vi "FindTopAndBottomEdges (SubVI).vi"(0 "Calibrated Image Array":T3[](array[typedef]), 1 "Fit Options":T7={"Number of Lines"=1, "Type"=enum."First Edge Rake", "Min. Score"=10.0, "Max. Score"=1000.0, "Orientation"=0.0, "Angle Range"=45.0, "Angle Tolerance"=1.0, "Step Size"=196, "Min. SNR (db)"=0.0, "Min. Points (%)"=25.0, "Hough Iterations"=5} {"Min. Points (%)" min=0.0 max=100.0; "Min. SNR (db)" min=0.0; "Max. Score" min=0.0 max=1024.0; "Min. Score" min=0.0 max=1024.0 step=1.0}, 5 "Options: Top Edge Search":T6={"Search Direction"=2, "Edge Options"={"Edge Polarity"=0, "Kernel Size"=5, "Width"=3, "Minimum Edge Strength"=16.0, "Interpolation Type"=enum."Bilinear Fixed", "Data Processing Method"=enum."Average"}, "Show Search Area"=TRUE, "Show Search Lines"=TRUE, "Show Edges Found"=TRUE, "Show Result"=TRUE, "Search Area Color"=65280, "Search Lines Color"=255, "Edge Locations Color"=16776960, "Result Color"=16711680, "Overlay Group Name"=""} {"Search Direction" items=["Left to Right", "Right to Left", "Top to Bottom", "Bottom to Top"]; "Edge Options"."Edge Polarity" items=["All Edges", "Rising Edges", "Falling Edges"]; "Edge Options"."Minimum Edge Strength" format="%.2f"; "Edge Options"."Width" step=2; "Edge Options"."Kernel Size" step=2}, 9 "Options: Bottom Edge Search":T6={"Search Direction"=3, "Edge Options"={"Edge Polarity"=2, "Kernel Size"=9, "Width"=3, "Minimum Edge Strength"=17.0, "Interpolation Type"=enum."Bilinear Fixed", "Data Processing Method"=enum."Average"}, "Show Search Area"=TRUE, "Show Search Lines"=TRUE, "Show Edges Found"=TRUE, "Show Result"=TRUE, "Search Area Color"=65280, "Search Lines Color"=255, "Edge Locations Color"=16776960, "Result Color"=16711680, "Overlay Group Name"=""} {"Search Direction" items=["Left to Right", "Right to Left", "Top to Bottom", "Bottom to Top"]; "Edge Options"."Edge Polarity" items=["All Edges", "Rising Edges", "Falling Edges"]; "Edge Options"."Minimum Edge Strength" format="%.2f"; "Edge Options"."Width" step=2; "Edge Options"."Kernel Size" step=2}, 11 "error in (no error)":errorcluster) -> (4 "Analyzed Image Array":T3[](array[typedef]), 6 "Top Edges":T1(array[cluster]), 8 "Bottom Edges":T1(array[cluster]), 10 "Array of Edge Endpoint Arrays":sgl[][][](array[numeric]), 15 "error out":errorcluster)   [LabVIEW 2016]
uses:
  <vilib>/vision/Measure.llb/Straight Edge Options.ctl
  <vilib>/vision/Measure.llb/Straight Edge Process.ctl
  <vilib>/vision/Measure.llb/Edge Options.ctl
  <vilib>/vision/Measure.llb/Edge Polarity.ctl
  <vilib>/vision/Image Controls.llb/IMAQ Image.ctl
  <vilib>/vision/NI_Vision_Development_Module.lvlib
panel:
  in  "ROI Descriptor - BOTTOM":T2={"Global Rectangle"=[0, 898, 2592, 1846], "Contours"=[{"ID"=enum."External", "Type"=12, "Coordinates"=[2, 898, 2591, 1846, 0]}]} {"Contours"."Type" items=["No Selection", "Point", "Line", "Rectangle", "Oval", "Polygon", "Freehand Region", "Annulus", "Unused2", "Unused3", "Broken Line", "Freehand Line", "Rotated Rectangle"]}
  in  "ROI Descriptor - TOP":T2={"Global Rectangle"=[0, 132, 2592, 1180], "Contours"=[{"ID"=enum."External", "Type"=12, "Coordinates"=[5, 132, 2612, 1180, 0]}]} {"Contours"."Type" items=["No Selection", "Point", "Line", "Rectangle", "Oval", "Polygon", "Freehand Region", "Annulus", "Unused2", "Unused3", "Broken Line", "Freehand Line", "Rotated Rectangle"]}
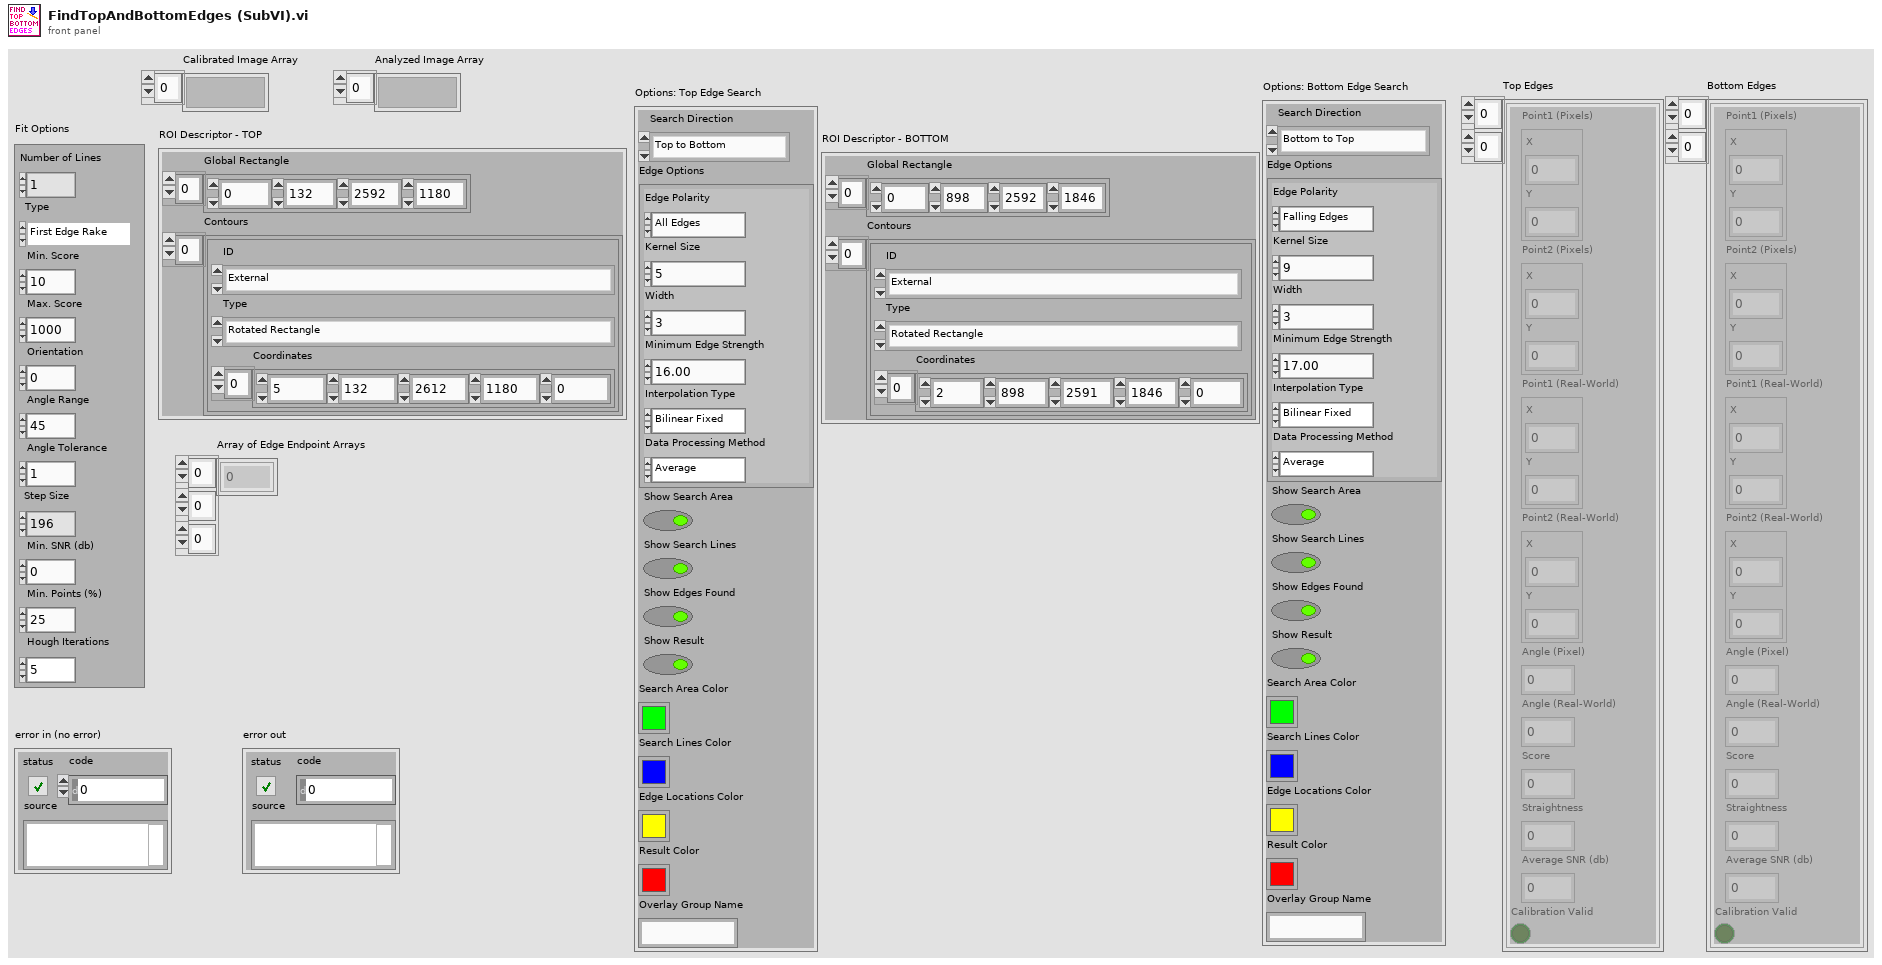
[diagram p1: front panel]
types:
  T1 = cluster{"Point1 (Pixels)":cluster{"X":sgl, "Y":sgl}, "Point2 (Pixels)":cluster{"X":sgl, "Y":sgl}, "Point1 (Real-World)":cluster{"X":sgl, "Y":sgl}, "Point2 (Real-World)":cluster{"X":sgl, "Y":sgl}, "Angle (Pixel)":dbl, "Angle (Real-World)":dbl, "Score":dbl, "Straightness":dbl, "Average SNR (db)":dbl, "Calibration Valid":bool}[][]
  T2 = cluster{"Global Rectangle":i32[], "Contours":cluster{"ID":enum32{"External", "Internal"}, "Type":u32, "Coordinates":i32[]}[]}
  T3 = typedef "IMAQ Image.ctl" = refnum<image>
  T4 = typedef "Edge Options.ctl" = cluster{"Edge Polarity":T5, "Kernel Size":u32, "Width":u32, "Minimum Edge Strength":sgl, "Interpolation Type":enum32{"Zero Order", "Bilinear", "Quadratic", "Cubic", "Bilinear Fixed"}, "Data Processing Method":enum32{"Average", "Median"}}
  T5 = typedef "Edge Polarity.ctl" = u32
  T6 = cluster{"Search Direction":u32, "Edge Options":T4, "Show Search Area":bool, "Show Search Lines":bool, "Show Edges Found":bool, "Show Result":bool, "Search Area Color":u32, "Search Lines Color":u32, "Edge Locations Color":u32, "Result Color":u32, "Overlay Group Name":string}
  T7 = typedef "Straight Edge Options.ctl" = cluster{"Number of Lines":i32, "Type":T8, "Min. Score":dbl, "Max. Score":dbl, "Orientation":dbl, "Angle Range":dbl, "Angle Tolerance":dbl, "Step Size":u32, "Min. SNR (db)":dbl, "Min. Points (%)":dbl, "Hough Iterations":i32}
  T8 = typedef "Straight Edge Process.ctl" = enum32{"First Edge Rake", "Best Edge Rake", "Hough Edge Rake", "First Edge Projection", "Best Edge Projection"}
  T9 = cluster{"Point1 (Pixels)":cluster{"X":sgl, "Y":sgl}, "Point2 (Pixels)":cluster{"X":sgl, "Y":sgl}, "Point1 (Real-World)":cluster{"X":sgl, "Y":sgl}, "Point2 (Real-World)":cluster{"X":sgl, "Y":sgl}, "Angle (Pixel)":dbl, "Angle (Real-World)":dbl, "Score":dbl, "Straightness":dbl, "Average SNR (db)":dbl, "Calibration Valid":bool}[]
  T10 = cluster{"Point1 (Pixels)":cluster{"X":sgl, "Y":sgl}, "Point2 (Pixels)":cluster{"X":sgl, "Y":sgl}, "Point1 (Real-World)":cluster{"X":sgl, "Y":sgl}, "Point2 (Real-World)":cluster{"X":sgl, "Y":sgl}, "Angle (Pixel)":dbl, "Angle (Real-World)":dbl, "Score":dbl, "Straightness":dbl, "Average SNR (db)":dbl, "Calibration Valid":bool}
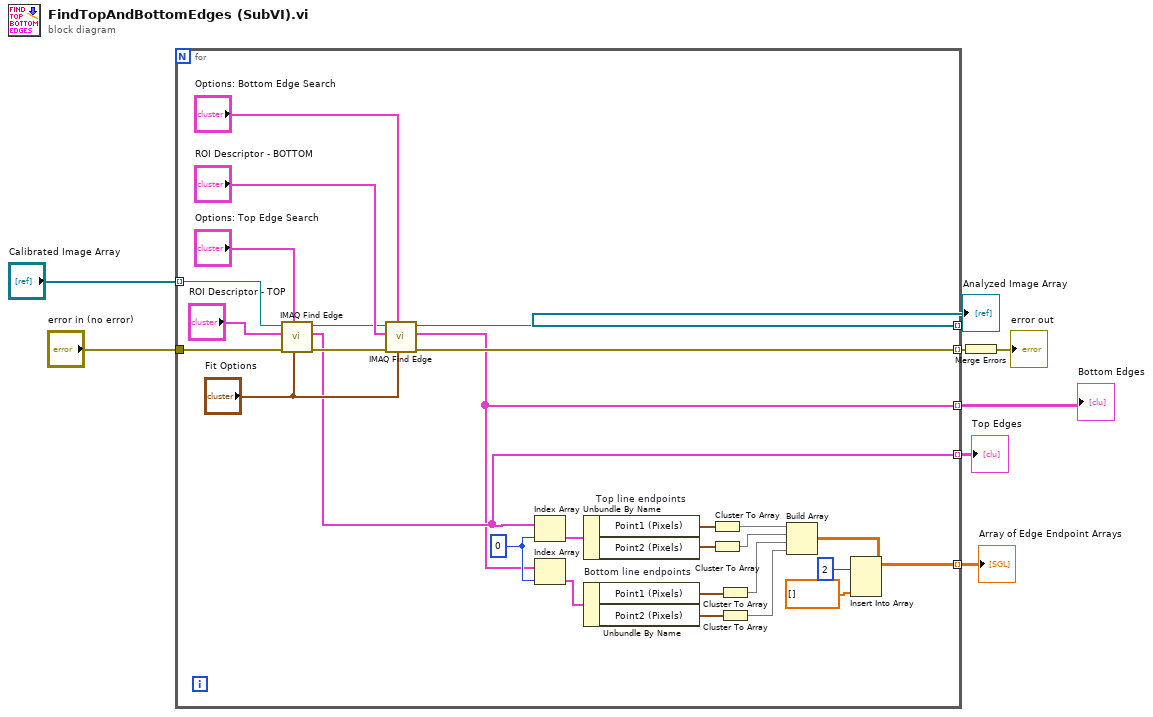
[diagram p0: block diagram]
diagram:
  n1 = for {
    tunnel: "Calibrated Image Array" -> [w36] mode=indexing
    tunnel: "error in (no error)" -> [w31]
    tunnel: [w30] -> w5 mode=indexing
    tunnel: [w28] -> w8 mode=indexing
    tunnel: [w11] -> w3 mode=indexing
    tunnel: [w10] -> w2 mode=indexing
    tunnel: [w9] -> w1 mode=indexing
    w25 = 0 ("index")
    n2 = call "IMAQ Find Edge"("Line Fit Options"="Fit Options", "Options"="Options: Top Edge Search", "error in (no error)"=w31, "ROI Descriptor"="ROI Descriptor - TOP", "Image"=w36) -> ("error out"=w26:errorcluster, "Straight Edges"=w11:T9, "Image Out"=w27:T3)  [unwired: 3 in, 1 out]
    n3 = call "IMAQ Find Edge"("Line Fit Options"="Fit Options", "Options"="Options: Bottom Edge Search", "error in (no error)"=w26, "ROI Descriptor"="ROI Descriptor - BOTTOM", "Image"=w27) -> ("error out"=w30:errorcluster, "Straight Edges"=w10:T9, "Image Out"=w28:T3)  [unwired: 3 in, 1 out]
    n4 = Index Array(array=w11, index=w25) -> (element=w24:T10)
    n5 = Index Array(array=w10, index=w25) -> (element=w23:T10)
    n6 = Unbundle By Name "Top line endpoints"(w24) -> ("Point1 (Pixels)"=w22:cluster{"X":sgl, "Y":sgl}, "Point2 (Pixels)"=w21:cluster{"X":sgl, "Y":sgl})
    n7 = Unbundle By Name "Bottom line endpoints"(w23) -> ("Point1 (Pixels)"=w14:cluster{"X":sgl, "Y":sgl}, "Point2 (Pixels)"=w15:cluster{"X":sgl, "Y":sgl})
    n8 = Cluster To Array(cluster=w22) -> (array=w20:sgl[])
    n9 = Cluster To Array(cluster=w21) -> (array=w19:sgl[])
    n10 = Cluster To Array(cluster=w14) -> (array=w13:sgl[])
    n11 = Cluster To Array(cluster=w15) -> (array=w12:sgl[])
    n12 = Build Array(w20, w19, w13, w12) -> (w18:sgl[][])
    n13 = Insert Into Array(array=w18, index (col)=2 ("disabled index (col)"), new element=sgl[] [] ("new element/subarray")) -> (w9:sgl[][])  [unwired: 1 in]
  }
  "Analyzed Image Array" <- w8
  "Top Edges" <- w3
  "Bottom Edges" <- w2
  "Array of Edge Endpoint Arrays" <- w1
  n14 = Merge Errors(w5) -> (→"error out":errorcluster)
